vi "Write Configuration Path.vi"(8 "error in (no error)":errorcluster, 10 "name or relative path":string, 11 "Instrument in":refnum<class "Instrument.lvclass">) -> (0 "error out":errorcluster, 3 "Instrument out":refnum<class "Instrument.lvclass">)   [LabVIEW 2019, in "Instrument.lvlib" / "Instrument.lvclass"]
uses:
  Instrument.lvclass
  Instrument.lvclass/Instrument.ctl
  <userlib>/LevyLab/Configuration/Configuration.lvclass
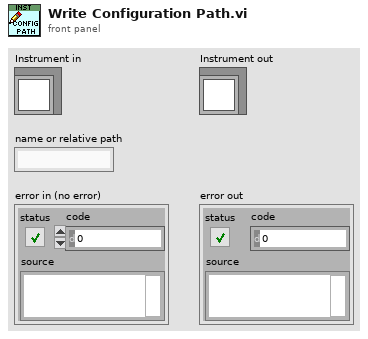
[diagram p1: front panel]
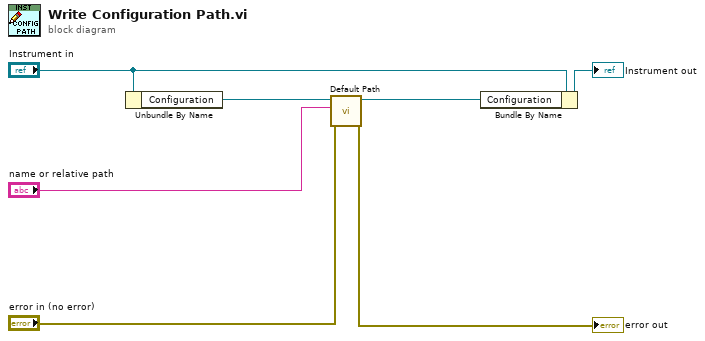
[diagram p0: block diagram]
diagram:
  n1 = Unbundle By Name("Instrument in") -> ("Configuration"=w5:refnum<class "Configuration.lvclass">)
  n2 = call <userlib>:"Default Path.vi"("error in (no error)"="error in (no error)", "Folder Name [Application Name]"="name or relative path", "Configuration in"=w5) -> ("error out"=→"error out":errorcluster, "Configuration out"=w2:refnum<class "Configuration.lvclass">)  [unwired: 7 in]
  n3 = Bundle By Name(cluster="Instrument in", "Configuration"=w2) -> (→"Instrument out":refnum<class "Instrument.lvclass">)
